vi "波形图类移动鼠标坐标显示.vi"() -> ()   [LabVIEW 2017]
panel:
  out "坐标":cluster{"X":dbl, "Y":dbl} {"Y" format="%.3f"; "X" format="%.3f"}
  out "XY图":cluster{i32[], dbl[]}(graph)
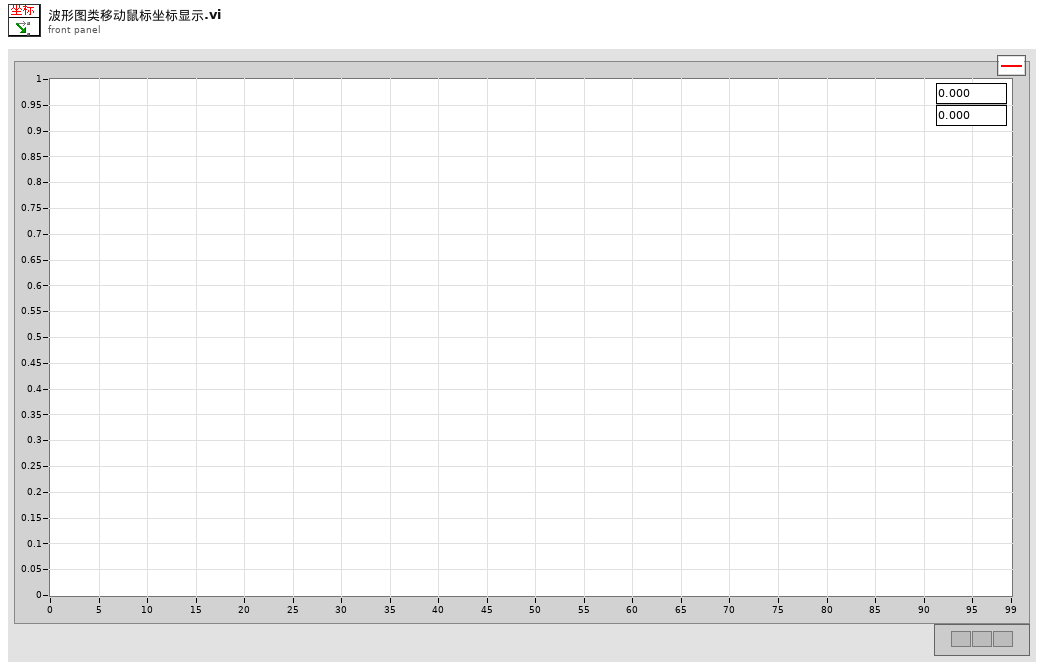
[diagram p1: front panel]
types:
  T1 = typedef "LVPoint32TypeDef.ctl" = cluster{"Horizontal":i32, "Vertical":i32}
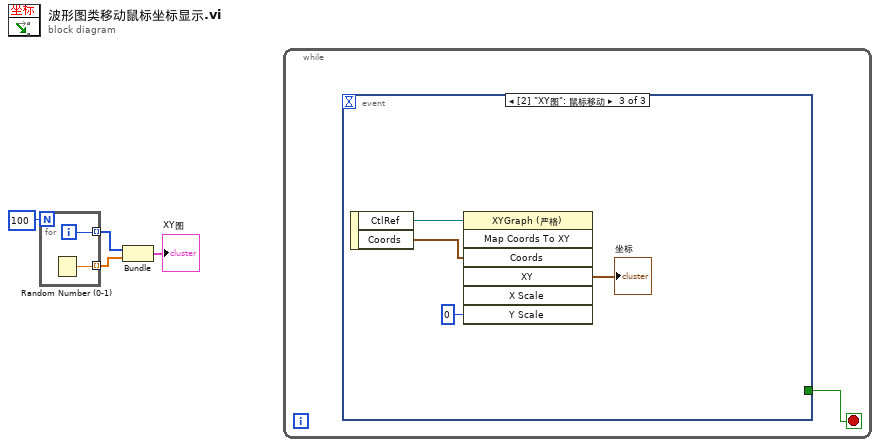
[diagram p0: block diagram]
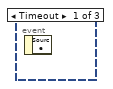
[diagram p2: hidden frame]
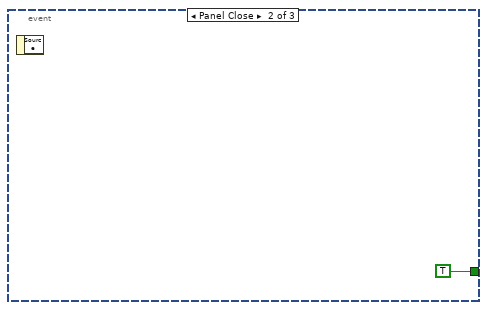
[diagram p3: hidden frame]
diagram:
  n1 = for {
    N: 100 -> [_]
    tunnel: [w6] -> w1 mode=indexing
    tunnel: [w5] -> w2 mode=indexing
    i -> [w5]
    n2 = Random Number (0-1)() -> (number: 0 to 1=w6:dbl)
  }
  n3 = Bundle(w2, w1) -> (→"XY图":cluster{i32[], dbl[]})  [unwired: 1 in]
  n4 = while {
    stop <- w7 stop-if-true
    n5 = event shown="[2] \"XY图\": 鼠标移动" {
      selector: _ -> [_ _ _]
      dyn-events: _ -> [_ _ _]
      timeout: _ -> [_ _ _]
      tunnel: [_ TRUE _] -> w7
      event Timeout {
        n6 = event-data() -> ()  [unwired: 1 in, 1 out]
      }
      event Panel Close {
        n7 = event-data() -> ()  [unwired: 1 in, 1 out]
      }
      event "XY图": Mouse Move {
        n8 = event-data() -> ("CtlRef"=w12:refnum<vi>, "Coords"=w11:T1)  [unwired: 1 in]
        n9 = invoke class="XYGraph (严格)" method="Map Coords To XY"(reference=w12, "Coords"=w11, "Y Scale"=0 ("Y标尺")) -> ("XY"=→"坐标":cluster{"X":dbl, "Y":dbl})  [unwired: 4 in, 6 out]
      }
    }
  }
